vi "03 Flow Meter Comparison Test SM.vi"() -> ()   [LabVIEW 2009]
uses:
  EquipReferences.ctl
  <vilib>/Utility/config.llb/Write Key (String).vi
  Intellifaucet/Intellfaucet Mode.ctl
  ChannelSettings.ctl
  <vilib>/Utility/config.llb/NI_LVConfig.lvlib
panel:
  in  "First Time":bool=TRUE
  out "XY Graph 3":T1(graph)
  in  "Automatic?":bool
  in  "Flow":i32
  in  "Offset(B)":dbl[](array[numeric])=[0.0, 0.0, 0.0]
  in  "Gain(m)":dbl[](array[numeric])=[1.0, 2.5, 1.0]
  out "Array":dbl[][](array[numeric])
  out "FLOW,34,35":dbl[](array[numeric])
  in  "mS between Samplse":u32=1000
  in  "Percent Open Test Data":i32[](array[numeric])=[0, 15, 20, 30, 40, 50, 60, 70, 80, 90, 100]
  out "Save Triger":i32
  in  "Config File Path":path=path "C:/NI-2010/Trunk/Hybrid Water Heater/HEWH First Hour Rating.ini"
  out "Percent Input":i32
  in  "Num Samples at Each Set Point":u32=20
  out "Results(Flow,Percent)":dbl[][](array[numeric])
  in  "Equipment":T2={"COM Port"="COM1", "MW100"="MW100", "AG34970"="A-34972A", "Chamber"="WT500"}
  in  "Semiphore":T3
  out "Error Out":errorcluster
  in  "Error In":errorcluster
  # "Mag, Turbine, Coriolis"
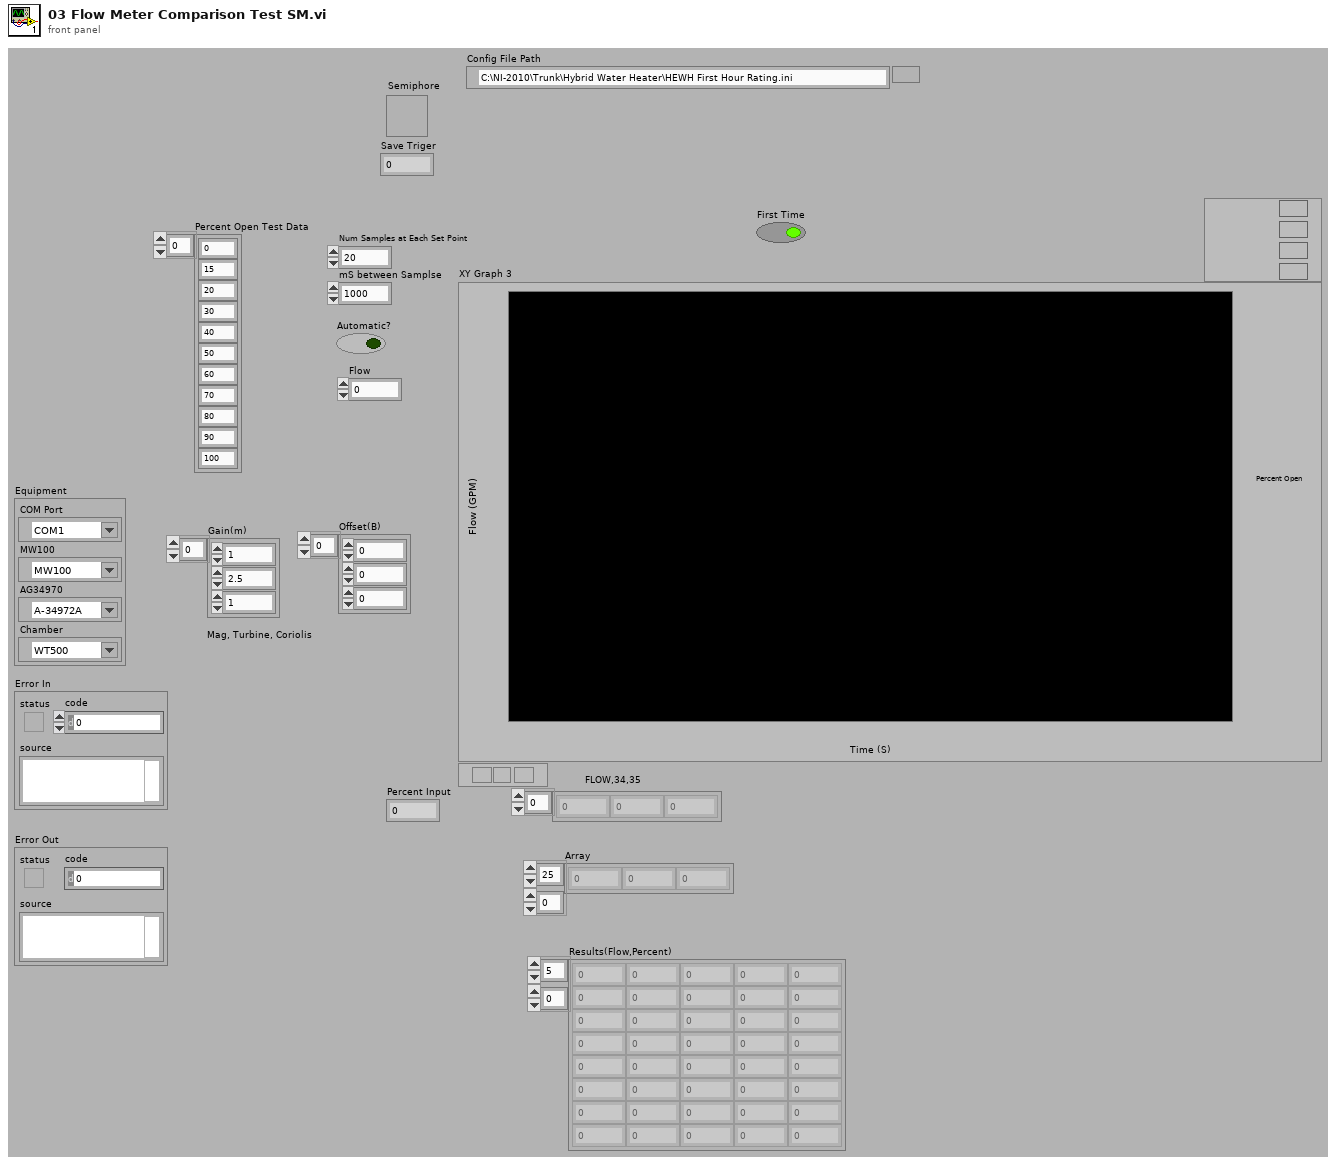
[diagram p1: front panel]
types:
  T1 = cluster{"XY chart data":cluster{"x":dbl, "y":dbl}[]}[]
  T2 = typedef "EquipReferences.ctl" = cluster{"COM Port":refnum<visa-resource-name>, "MW100":refnum<visa-resource-name>, "AG34970":refnum<visa-resource-name>, "Chamber":refnum<visa-resource-name>}
  T3 = typedef "Semaphore RefNum" = refnum<k1>
  T4 = typedef "Intellfaucet Mode.ctl" = enum16{"Adjust Temp", "Adjust Flow", "Start Flow", "Stop Flow"}
  T5 = cluster{cluster{"Elapsed Time (sec)":dbl, "Value":dbl}[]}[]
  T6 = typedef "NI_LVConfig.lvlib/Config Data RefNum.ctl" = refnum<k1>
  T7 = typedef "ChannelSettings.ctl" = u32
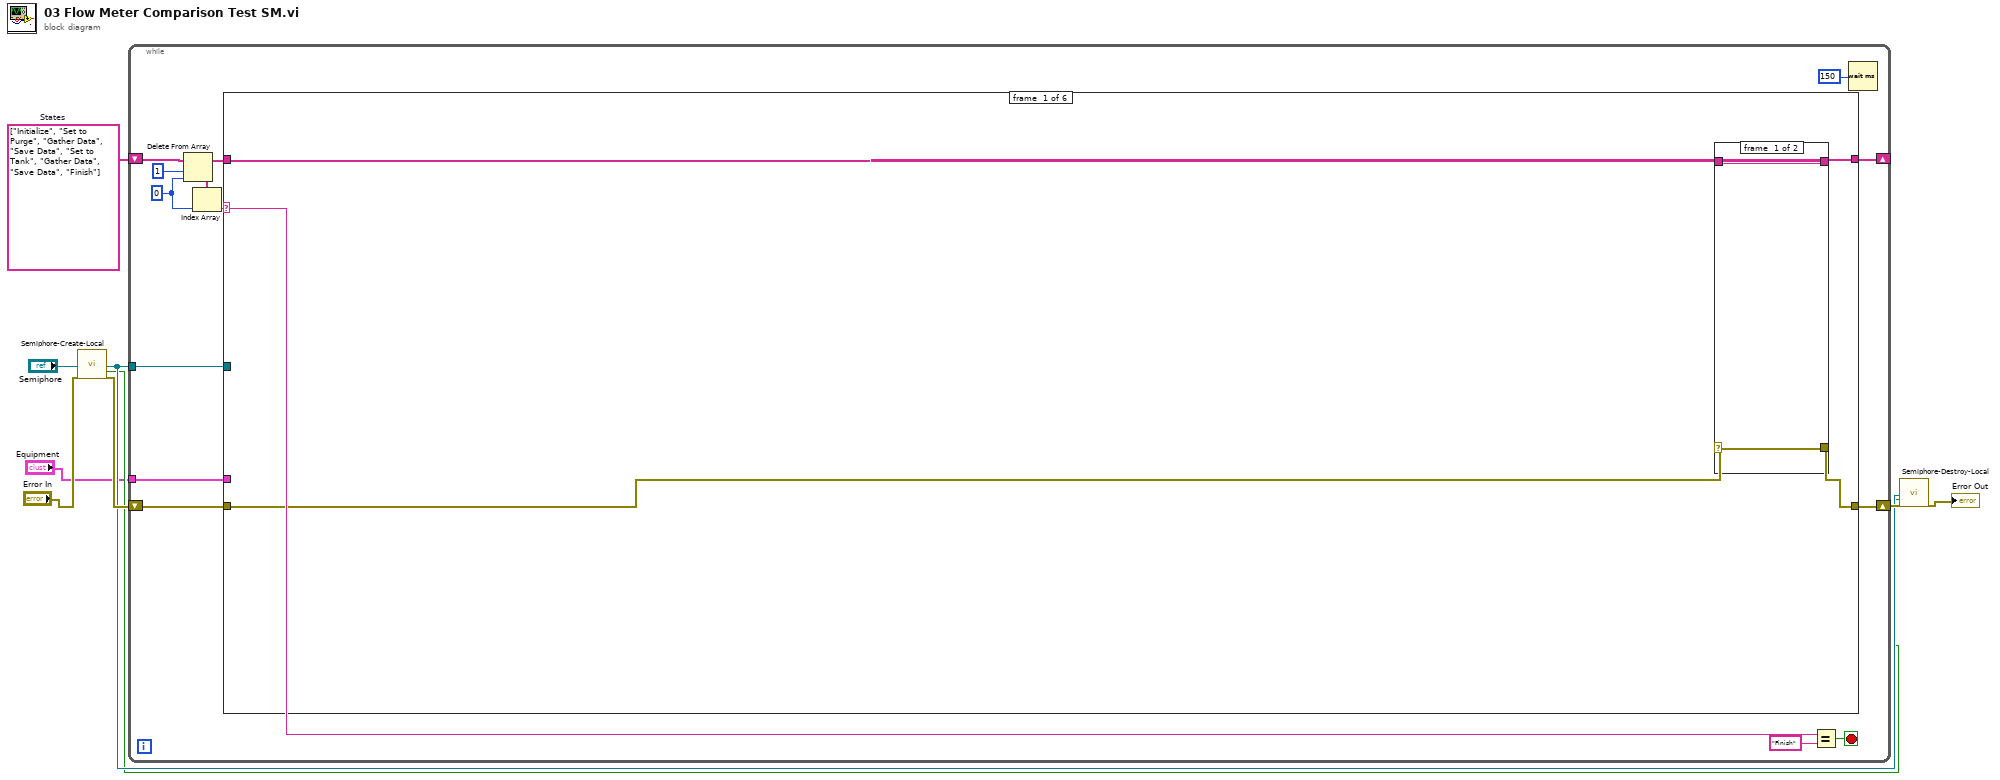
[diagram p0: block diagram]
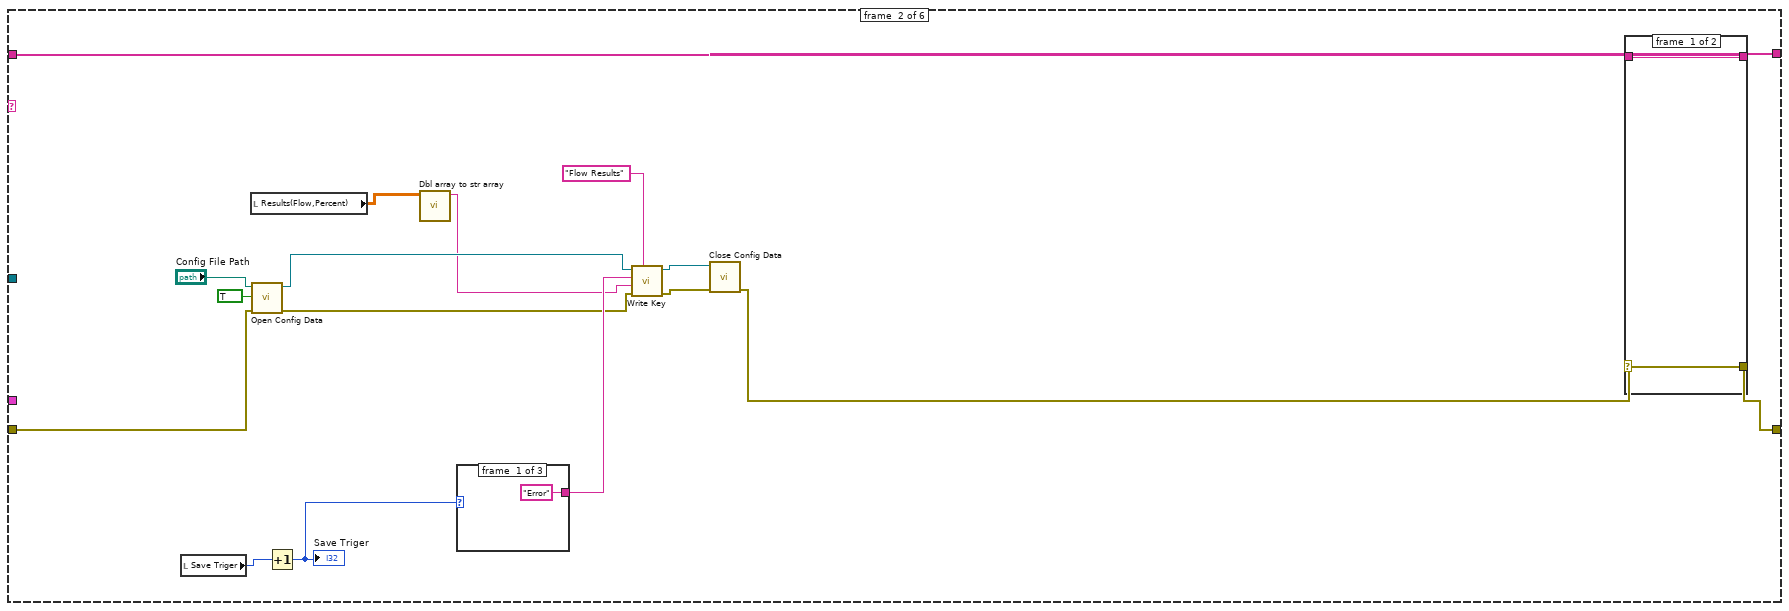
[diagram p3: hidden frame]
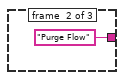
[diagram p4: hidden frame]
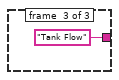
[diagram p5: hidden frame]
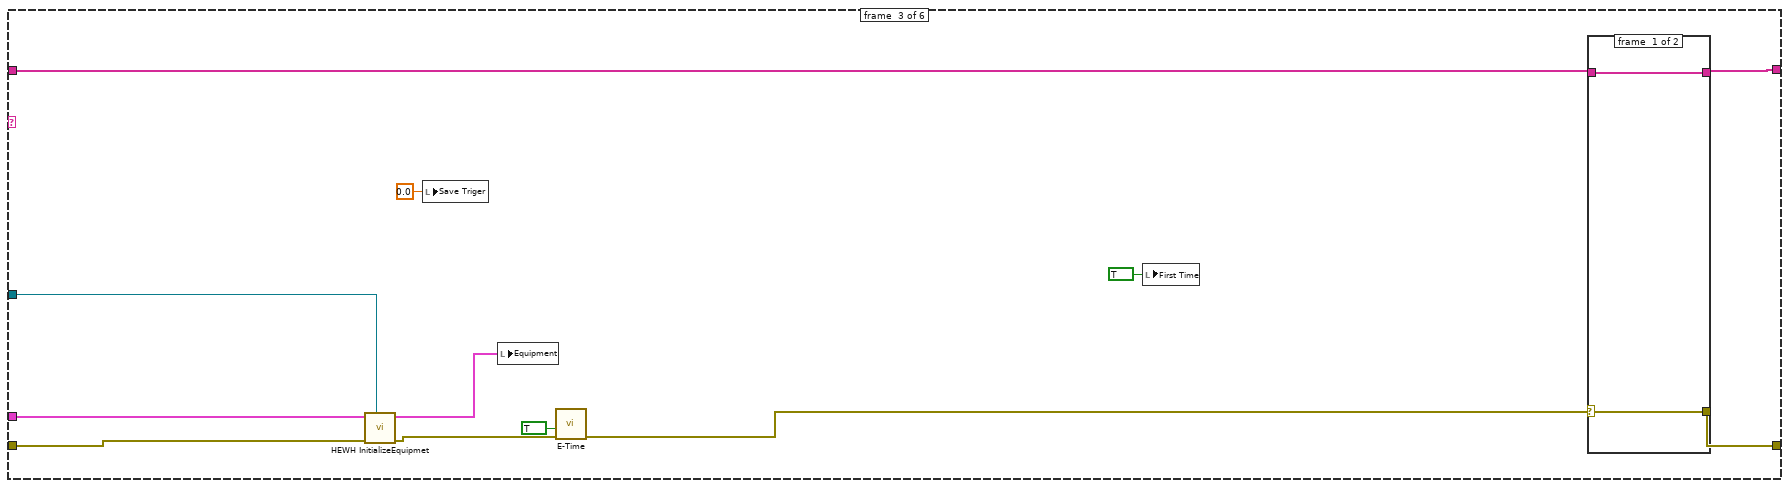
[diagram p7: hidden frame]
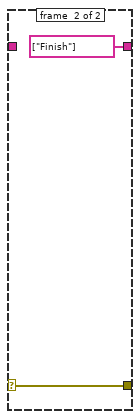
[diagram p8: hidden frame]
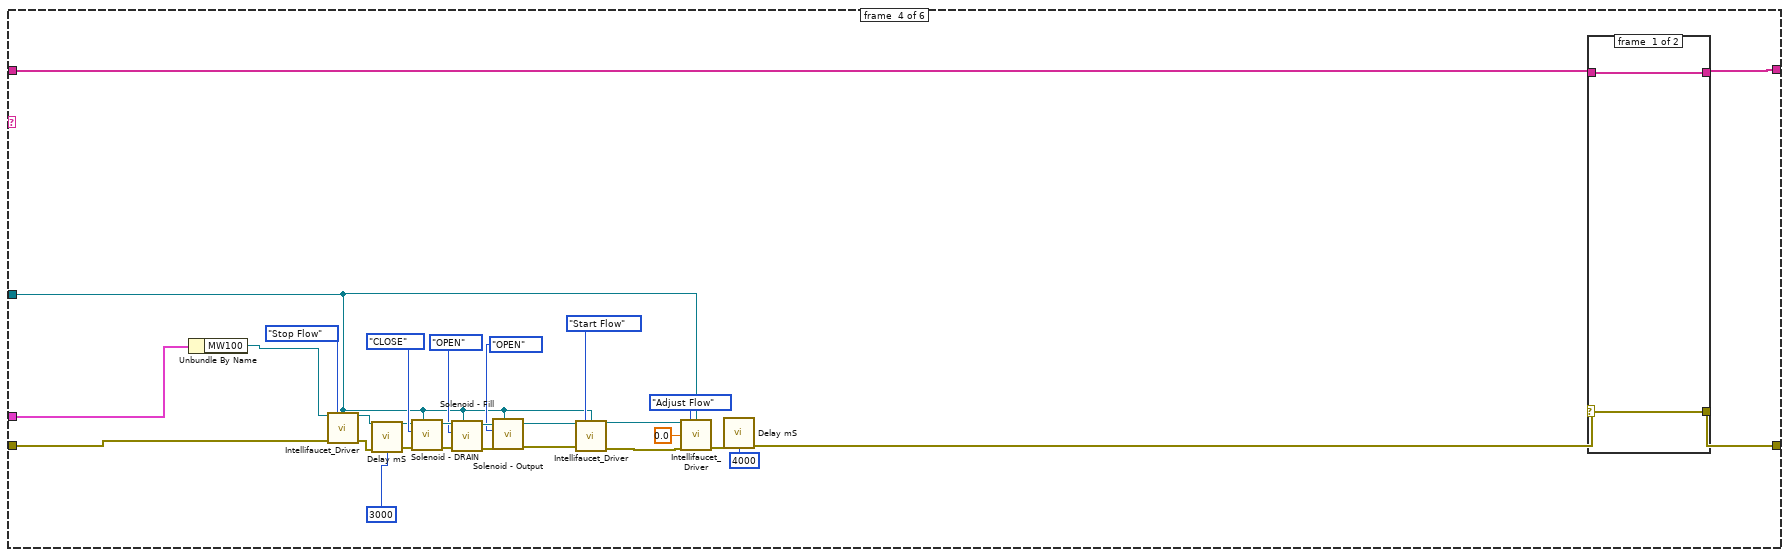
[diagram p9: hidden frame]
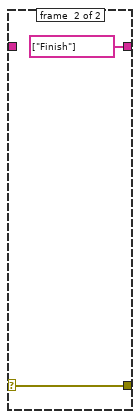
[diagram p10: hidden frame]
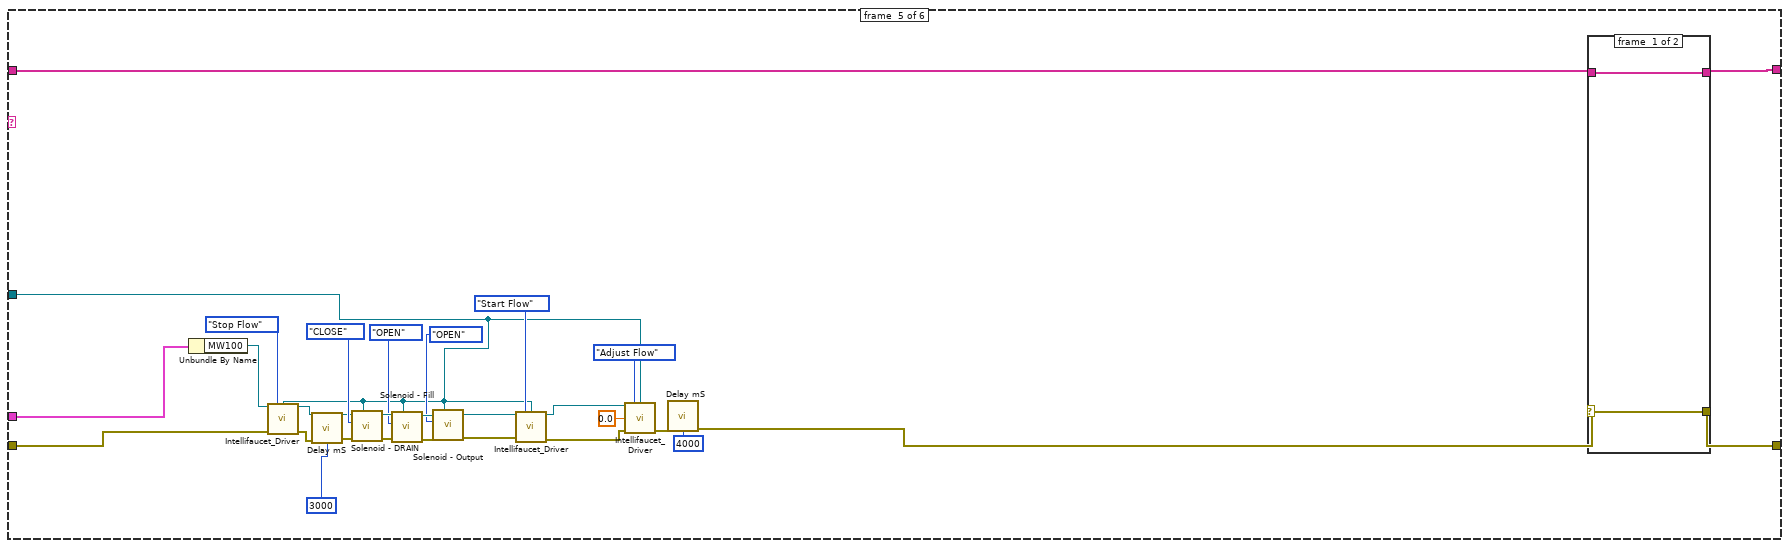
[diagram p11: hidden frame]
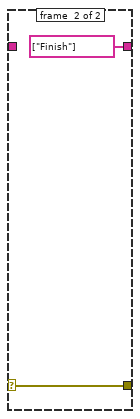
[diagram p12: hidden frame]
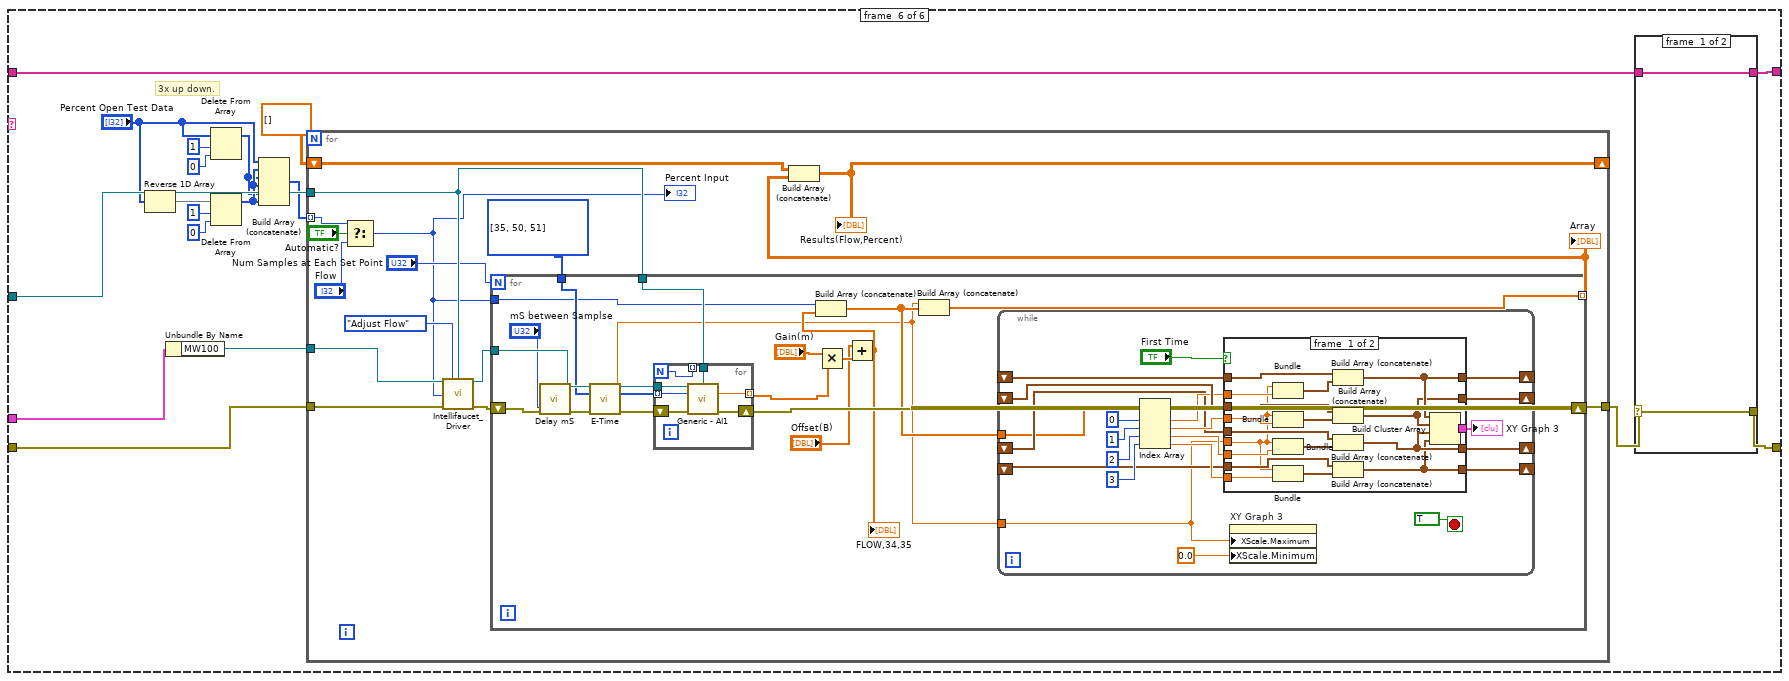
[diagram p13: hidden frame]
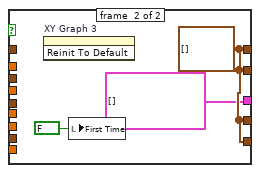
[diagram p14: hidden frame]
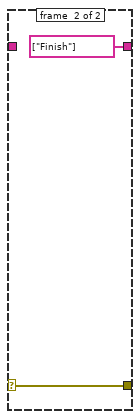
[diagram p15: hidden frame]
diagram:
  w9 = string[] ["Initialize", "Set to Purge", "Gather Data", "Save Data", "Set to Tank", "Gather Data", "Save Data", "Finish"]  # States
  n1 = call "Semiphore-Create-Local.vi"("Semiphore"="Semiphore", "error in (no error)"="Error In") -> ("semaphore"=w3:T3, "Local?"=w2:bool, "error out"=w6:errorcluster)  [unwired: 15 in]
  n2 = while {
    shift-right: [w19] -> _
    shift-left: w9 -> [w23]
    shift-right: [w16] -> w5
    shift-left: w6 -> [w15]
    tunnel: w3 -> [w11]
    tunnel: "Equipment" -> [w10]
    stop <- w14 stop-if-true
    w20 = 0 ("index")
    n3 = Delete From Array(array=w23, length=1, index=w20) -> (deleted portion=w21:string[], array with subset deleted=w18:string[])
    n4 = Index Array(array=w21, index=w20) -> (element=w13:string)
    n5 = case shown="\"Gather Data\"" w13 {
      tunnel: [w27 w48 w61 w98 w131 w153] -> w19
      tunnel: w18 -> [w26 w47 w62 w99 w132 w154]
      tunnel: [w25 w46 w63 w100 w133 w155] -> w16
      tunnel: w15 -> [w24 w37 w67 w82 w115 w150]
      tunnel: w11 -> [_ _ w66 w72 w108 w148]
      tunnel: w10 -> [_ _ w64 w81 w114 w152]
      frame #0 {
        n6 = case shown="Error" w24 {
          selector: w24 -> [w28 w30]
          tunnel: [w29 w31] -> w27
          tunnel: w26 -> [w29 w31]
          tunnel: [w28 w30] -> w25
          frame #0 {
          }
          frame #1 {
          }
        }
      }
      frame #1 {
        n7 = local read "Save Triger"() -> (w32:i32)
        n8 = local read "Results(Flow,Percent)"() -> (w45:dbl[][])
        n9 = call <vilib>:"Open Config Data.vi"("error in (no error)"=w37, "create file if necessary (T)"=TRUE, "configuration file path"="Config File Path") -> ("error out"=w40:errorcluster, "refnum"=w42:T6)  [unwired: 7 out]
        n10 = Increment(x=w32) -> (x+1=w33:i32)
        "Save Triger" <- w33
        n11 = call "Dbl array to str array.vi"("Array in"=w45) -> ("String array out"=w34:string)  [unwired: 9 in, 1 out]
        n12 = case shown="0, Default" w33 {
          tunnel: ["Error" ("key") "Purge Flow" ("key") "Tank Flow" ("key")] -> w41
          frame #0 {
          }
          frame #1 {
          }
          frame #2 {
          }
        }
        n13 = call-poly <vilib>:"Write Key.vi"("section"="Flow Results", "error in (no error)"=w40, "value"=w34, "key"=w41, "refnum"=w42) -> ("error out"=w39:errorcluster, "refnum out"=w38:T6)  [unwired: 1 in, 4 out]
        n14 = call <vilib>:"Close Config Data.vi"("error in (no error)"=w39, "refnum"=w38) -> ("error out"=w36:errorcluster)  [unwired: 1 in, 8 out]
        n15 = case shown="Error" w36 {
          selector: w36 -> [w52 w54]
          tunnel: [w53 w55] -> w48
          tunnel: w47 -> [w53 w55]
          tunnel: [w52 w54] -> w46
          frame #0 {
          }
          frame #1 {
          }
        }
      }
      frame #2 {
        n16 = call "HEWH InitializeEquipmet.vi"("Semiphore"=w66, "Error In"=w67, "Equipment"=w64) -> ("Error Out"=w59:errorcluster, "Equipment Out"=w65:T2)  [unwired: 5 in, 2 out]
        n17 = local write "Save Triger"(0.0 ("Save Triger")) -> ()
        n18 = local write "Equipment"(w65) -> ()
        n19 = call "E-Time.vi"("error in (no error)"=w59, "Reset"=TRUE) -> ("error out"=w58:errorcluster)  [unwired: 7 in, 2 out]
        n20 = local write "First Time"(TRUE ("First Time")) -> ()
        n21 = case shown="No Error" w58 {
          selector: w58 -> [w68 w71]
          tunnel: [w69 string[] ["Finish"] ("States")] -> w61
          tunnel: w62 -> [w69 _]
          tunnel: [w68 w71] -> w63
          frame #0 {
          }
          frame #1 {
          }
        }
      }
      frame #3 {
        n22 = Unbundle By Name(w81) -> ("MW100"=w80:refnum<visa-resource-name>)
        n23 = call "Intellifaucet_Driver.vi"("VISA session"=w80, "Mode"=Intellfaucet_Mode."Stop Flow", "Semiphore"=w72, "Error In"=w82) -> ("VISA session out"=w89:refnum<visa-resource-name>, "Error Out"=w88:errorcluster)  [unwired: 10 in]
        n24 = call "Delay mS.vi"("Error In"=w88, "milliseconds to wait"=u32 3000) -> ("Error Out"=w87:errorcluster)  [unwired: 13 in]
        n25 = call "Solenoid - DRAIN.vi"("Semiphore"=w72, "Error In"=w87, "VALVE OPEN CLOSE"=enum8{"OPEN", "CLOSE"}."CLOSE", "VISA session"=w89) -> ("Error Out"=w97:errorcluster, "dup VISA session"=w96:refnum<visa-resource-name>)  [unwired: 6 in]
        n26 = call "Solenoid - Fill.vi"("Semiphore"=w72, "Error In"=w97, "VALVE OPEN CLOSE"=enum8{"OPEN", "CLOSE"}."OPEN" ("OPEN CLOSE"), "VISA session"=w96) -> ("Error Out"=w94:errorcluster, "dup VISA session"=w93:refnum<visa-resource-name>)  [unwired: 6 in]
        n27 = call "Solenoid - Output.vi"("Semiphore"=w72, "Error In"=w94, "OPEN CLOSE"=enum8{"CLOSE", "OPEN"}."OPEN", "VISA session"=w93) -> ("Error Out"=w83:errorcluster, "dup VISA session"=w90:refnum<visa-resource-name>)  [unwired: 6 in]
        n28 = call "Intellifaucet_Driver.vi"("VISA session"=w90, "Mode"=Intellfaucet_Mode."Start Flow", "Semiphore"=w72, "Error In"=w83) -> ("VISA session out"=w73:refnum<visa-resource-name>, "Error Out"=w75:errorcluster)  [unwired: 10 in]
        n29 = call "Intellifaucet_Driver.vi"("VISA session"=w73, "Mode"=Intellfaucet_Mode."Adjust Flow", "Semiphore"=w72, "Percent Flow"=0.0, "Error In"=w75) -> ("Error Out"=w77:errorcluster)  [unwired: 9 in, 1 out]
        n30 = call "Delay mS.vi"("Error In"=w77, "milliseconds to wait"=u32 4000) -> ("Error Out"=w74:errorcluster)  [unwired: 13 in]
        n31 = case shown="Error" w74 {
          selector: w74 -> [w101 w104]
          tunnel: [w102 string[] ["Finish"] ("States")] -> w98
          tunnel: w99 -> [w102 _]
          tunnel: [w101 w104] -> w100
          frame #0 {
          }
          frame #1 {
          }
        }
      }
      frame #4 {
        n32 = Unbundle By Name(w114) -> ("MW100"=w113:refnum<visa-resource-name>)
        n33 = call "Intellifaucet_Driver.vi"("VISA session"=w113, "Mode"=Intellfaucet_Mode."Stop Flow", "Semiphore"=w108, "Error In"=w115) -> ("VISA session out"=w122:refnum<visa-resource-name>, "Error Out"=w121:errorcluster)  [unwired: 10 in]
        n34 = call "Delay mS.vi"("Error In"=w121, "milliseconds to wait"=u32 3000) -> ("Error Out"=w120:errorcluster)  [unwired: 13 in]
        n35 = call "Solenoid - DRAIN.vi"("Semiphore"=w108, "Error In"=w120, "VALVE OPEN CLOSE"=enum8{"OPEN", "CLOSE"}."CLOSE", "VISA session"=w122) -> ("Error Out"=w130:errorcluster, "dup VISA session"=w129:refnum<visa-resource-name>)  [unwired: 6 in]
        n36 = call "Solenoid - Fill.vi"("Semiphore"=w108, "Error In"=w130, "VALVE OPEN CLOSE"=enum8{"OPEN", "CLOSE"}."OPEN" ("OPEN CLOSE"), "VISA session"=w129) -> ("Error Out"=w127:errorcluster, "dup VISA session"=w126:refnum<visa-resource-name>)  [unwired: 6 in]
        n37 = call "Solenoid - Output.vi"("Semiphore"=w108, "Error In"=w127, "OPEN CLOSE"=enum8{"CLOSE", "OPEN"}."OPEN", "VISA session"=w126) -> ("Error Out"=w116:errorcluster, "dup VISA session"=w123:refnum<visa-resource-name>)  [unwired: 6 in]
        n38 = call "Intellifaucet_Driver.vi"("VISA session"=w123, "Mode"=Intellfaucet_Mode."Start Flow", "Semiphore"=w108, "Error In"=w116) -> ("VISA session out"=w109:refnum<visa-resource-name>, "Error Out"=w110:errorcluster)  [unwired: 10 in]
        n39 = call "Intellifaucet_Driver.vi"("VISA session"=w109, "Mode"=Intellfaucet_Mode."Adjust Flow", "Semiphore"=w108, "Percent Flow"=0.0, "Error In"=w110) -> ("Error Out"=w107:errorcluster)  [unwired: 9 in, 1 out]
        n40 = call "Delay mS.vi"("Error In"=w107, "milliseconds to wait"=u32 4000) -> ("Error Out"=w106:errorcluster)  [unwired: 13 in]
        n41 = case shown="Error" w106 {
          selector: w106 -> [w134 w137]
          tunnel: [w135 string[] ["Finish"] ("States")] -> w131
          tunnel: w132 -> [w135 _]
          tunnel: [w134 w137] -> w133
          frame #0 {
          }
          frame #1 {
          }
        }
      }
      frame #5 {
        # "3x up down."
        n42 = Reverse 1D Array(array="Percent Open Test Data") -> (reversed array=w145:i32[])
        n43 = Unbundle By Name(w152) -> ("MW100"=w151:refnum<visa-resource-name>)
        n44 = Delete From Array(array="Percent Open Test Data", length=1, index=0) -> (array with subset deleted=w146:i32[])  [unwired: 1 out]
        n45 = Delete From Array(array=w145, length=1, index=0) -> (array with subset deleted=w147:i32[])  [unwired: 1 out]
        n46 = Build Array (concatenate)("Percent Open Test Data", w147, w146, w147, w146, w147) -> (w139:i32[])
        n47 = for {
          tunnel: w150 -> [w169]
          tunnel: w148 -> [w168]
          tunnel: [w171] -> w149
          tunnel: w139 -> [w159] mode=indexing
          tunnel: w151 -> [w165]
          shift-right: [w161] -> _
          shift-left: dbl[][] [] -> [w160]
          w163 = T7[] [35, 50, 51] items=["4-20_OUT", "Pres_HI1", "Pres_HI2", "Pres_LOW", "Pres_PIN", "HEATER_TOP", "HEATER_BOT", "T_Shell", "FLOWMETER", "WATT_SENSE", "WH_TICK", "Tc_1", "Tc_2", "Tc_3", "Tc_4", "Tc_5", "Tc_6", "Tc_down", "T_Shell_2", "T_Shell_3", "T_Shell_4", "RTD_IN", "RTD_OUT", "RTD_AMB", "INTF_TEMPFLO", "INTF_READY", "INTF_START", "INTF_STOP", "DRM_LOW", "DRM_HIGH", "PWR_MAIN", "VLV_DUMP", "VLV_OUT", "VLV_IN", "WATT_HOURS", "FLOW(SAMPLE)", "GALLONS", "FLOW(GPM)", "FLOW_CALC_GAIN", "FLOW_CALC_OFFSET", "FLOW_CALC_THRESHOLD", "VLV_DUMP_2", "VLV_OUT_2", "VLV_IN_2", "VLV_DUMP_3", "VLV_OUT_3", "VLV_IN_3", "VLV_DUMP_4", "VLV_OUT_4", "VLV_IN_4", "CHAN_34", "CHAN_35", "CHAN_36"]
          n48 = Select(t=w159, s="Automatic?", f="Flow") -> (s? t:f=w158:i32)
          "Percent Input" <- w158
          n49 = call "Intellifaucet_Driver.vi"("VISA session"=w165, "Mode"=Intellfaucet_Mode."Adjust Flow", "Semiphore"=w168, "Percent Flow"=w158, "Error In"=w169) -> ("VISA session out"=w166:refnum<visa-resource-name>, "Error Out"=w170:errorcluster)  [unwired: 9 in]
          n50 = for {
            N: "Num Samples at Each Set Point" -> [_]
            tunnel: w168 -> [w186]
            tunnel: w166 -> [w185]
            shift-right: [w188] -> w171
            shift-left: w170 -> [w187]
            tunnel: [w174] -> w162 mode=indexing
            tunnel: w163 -> [w183]
            tunnel: w158 -> [w180]
            n51 = call "Delay mS.vi"("Error In"=w187, "milliseconds to wait"="mS between Samplse") -> ("Error Out"=w182:errorcluster)  [unwired: 13 in]
            n52 = call "E-Time.vi"("error in (no error)"=w182) -> ("error out"=w181:errorcluster, "Elapsed Time (sec)"=w172:dbl)  [unwired: 8 in, 1 out]
            n53 = for {
              N -> [w232]
              tunnel: w183 -> [w238] mode=indexing
              tunnel: w186 -> [w235]
              tunnel: w185 -> [w234]
              tunnel: [w233] -> w177 mode=indexing
              shift-right: [w236] -> w188
              shift-left: w181 -> [w237]
              tunnel: [w232] -> _ mode=indexing
              n54 = call "Generic - AI1.vi"("MW100"=w234, "Semiphore"=w235, "Channel_Enum"=w238, "Error In"=w237) -> ("Value"=w233:dbl, "Error Out"=w236:errorcluster)  [unwired: 9 in, 1 out]
            }
            n55 = Multiply(x="Gain(m)", y=w177) -> (x*y=w179:dbl[])
            n56 = Add(x="Offset(B)", y=w179) -> (x+y=w176:dbl[])
            "FLOW,34,35" <- w176
            n57 = Build Array (concatenate)(w180, w176) -> (w173:dbl[])
            n58 = Build Array (concatenate)(w172, w173) -> (w174:dbl[])
            n59 = while {
              shift-right: [w209] -> _
              shift-left: _ -> [w207]
              shift-right: [w208] -> _
              shift-left: _ -> [w206]
              shift-right: [w193] -> _
              shift-left: _ -> [w195]
              shift-right: [w192] -> _
              shift-left: _ -> [w194]
              tunnel: w172 -> [w191]
              tunnel: w173 -> [w190]
              stop <- TRUE ("stop") stop-if-true
              n60 = Index Array(array=w190, index #1=0 ("index"), index #2=1 ("index"), index #3=2 ("index"), index #4=3 ("index")) -> (element #1=w199:dbl, element #2=w198:dbl, element #3=w197:dbl, element #4=w196:dbl)
              n61 = case shown="True" "First Time" {
                tunnel: [w228 T5 []] -> w210
                tunnel: [w227 w231] -> w209
                tunnel: [w226 w231] -> w208
                tunnel: w207 -> [w225 _]
                tunnel: w206 -> [w224 _]
                tunnel: w199 -> [w223 _]
                tunnel: w198 -> [w222 _]
                tunnel: w197 -> [w221 _]
                tunnel: w196 -> [w220 _]
                tunnel: w195 -> [w219 _]
                tunnel: w194 -> [w218 _]
                tunnel: [w217 w231] -> w193
                tunnel: [w216 w231] -> w192
                tunnel: w191 -> [w215 _]
                frame #0 {
                  n62 = Bundle("Elapsed Time (sec)"=w215, "Value"=w223) -> (w214:cluster{"Elapsed Time (sec)":dbl, "Value":dbl})  [unwired: 1 in]
                  n63 = Bundle("Elapsed Time (sec)"=w215, "Value"=w222) -> (w213:cluster{"Elapsed Time (sec)":dbl, "Value":dbl})  [unwired: 1 in]
                  n64 = Bundle("Elapsed Time (sec)"=w215, "Value"=w221) -> (w212:cluster{"Elapsed Time (sec)":dbl, "Value":dbl})  [unwired: 1 in]
                  n65 = Bundle("Elapsed Time (sec)"=w215, "Value"=w220) -> (w211:cluster{"Elapsed Time (sec)":dbl, "Value":dbl})  [unwired: 1 in]
                  n66 = Build Array (concatenate)(w225, w214) -> (w227:cluster{"Elapsed Time (sec)":dbl, "Value":dbl}[])
                  n67 = Build Array (concatenate)(w224, w213) -> (w226:cluster{"Elapsed Time (sec)":dbl, "Value":dbl}[])
                  n68 = Build Array (concatenate)(w219, w212) -> (w217:cluster{"Elapsed Time (sec)":dbl, "Value":dbl}[])
                  n69 = Build Array (concatenate)(w218, w211) -> (w216:cluster{"Elapsed Time (sec)":dbl, "Value":dbl}[])
                  n70 = Build Cluster Array(w227, w226, w217, w216) -> (w228:T5)
                }
                frame #1 {
                  w231 = cluster{"Elapsed Time (sec)":dbl, "Value":dbl}[] []
                  n71 = invoke on="XY Graph 3" class="XYGraph (strict)" method="Reinit To Default"() -> ()  [unwired: 3 in, 3 out]
                  n72 = local write "First Time"(FALSE ("First Time")) -> ()
                }
              }
              "XY Graph 3" <- w210
              n73 = property on="XY Graph 3" class="XYGraph (strict)"("XScale.Maximum"=w191, "XScale.Minimum"=0.0 ("X Scale.Range:Minimum")) -> ()  [unwired: 2 in, 2 out]
            }
          }
          "Array" <- w162
          n74 = Build Array (concatenate)(w160, w162) -> (w161:dbl[][])
          "Results(Flow,Percent)" <- w161
        }
        n75 = case shown="Error" w149 {
          selector: w149 -> [w239 w242]
          tunnel: [w240 string[] ["Finish"] ("States")] -> w153
          tunnel: w154 -> [w240 _]
          tunnel: [w239 w242] -> w155
          frame #0 {
          }
          frame #1 {
          }
        }
      }
    }
    n76 = Equal?(x=w13, y="Finish") -> (x = y?=w14:bool)
    n77 = Wait (ms)(milliseconds to wait=u32 150) -> ()  [unwired: 1 out]
  }
  n78 = call "Semiphore-Destroy-Local.vi"("Semiphore"=w3, "Local?"=w2, "error in (no error)"=w5) -> ("error out"=→"Error Out":errorcluster)  [unwired: 16 in]
